vi "Template.vi"(11 "Interface in":refnum<class "Interface.lvclass">) -> ()   [LabVIEW 2021, in "Interface.lvclass"]
uses:
  Interface.lvclass
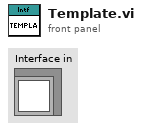
[diagram p1: front panel]
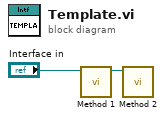
[diagram p0: block diagram]
diagram:
  n1 = call-dynamic "Method 1.vi"("Interface 1 in"="Interface in") -> ("Interface 1 out"=w1:refnum<class "Interface.lvclass">)  [unwired: 9 in, 1 out]
  n2 = call-dynamic "Method 2.vi"("Interface 2 in"=w1) -> ()  [unwired: 9 in, 2 out]
